vi "calculate binningMAGSPEC.vi"(10 "Value":dbl, 11 "Refnum in":T1) -> (3 "Numeric":dbl)   [LabVIEW 2011]
uses:
  <vilib>/vision/Image Controls.llb/IMAQ Image.ctl
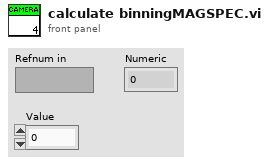
[diagram p1: front panel]
types:
  T1 = typedef "IMAQ Image.ctl" = refnum<image>
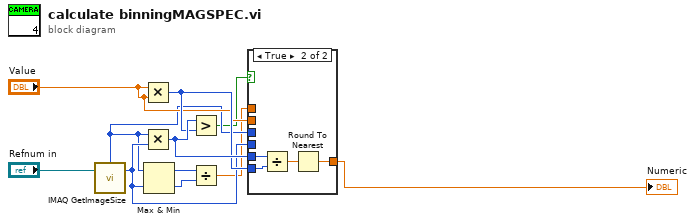
[diagram p0: block diagram]
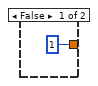
[diagram p2: hidden frame]
diagram:
  n1 = call "IMAQ GetImageSize"("Image"="Refnum in") -> ("Y Resolution"=w7:i32, "X Resolution"=w6:i32)  [unwired: 3 in, 1 out]
  n2 = Multiply(x="Value", y="Value") -> (x*y=w9:u64)
  n3 = Multiply(x=w6, y=w7) -> (x*y=w10:u64)
  n4 = Max & Min(x=w6, y=w7) -> (max(x,y)=w3:i32, min(x,y)=w1:i32)
  n5 = Greater?(x=w10, y=w9) -> (0:w4:bool)
  n6 = Divide(x=w3, y=w1) -> (x/y=w2:dbl)
  n7 = case shown="True" w4 {
    tunnel: w2 -> [_ _]
    tunnel: "Value" -> [_ _]
    tunnel: w6 -> [_ _]
    tunnel: w7 -> [_ _]
    tunnel: [1 w15] -> w5
    tunnel: w9 -> [_ w14]
    tunnel: w10 -> [_ w13]
    frame False {
    }
    frame True {
      n8 = Divide(x=w13, y=w14) -> (x/y=w16:dbl)
      n9 = Round To Nearest(number=w16) -> (nearest integer value=w15:dbl)
    }
  }
  "Numeric" <- w5
